vi "MS-200 Send Command.vi"(0 "VISA Ref":refnum<visa-resource-name>, 2 "Wait for Reply (T)":bool=TRUE, 7 "Command":string, 11 "Error In":errorcluster) -> (4 "VISA Ref Dup":refnum<visa-resource-name>, 8 "Reply":string, 13 "Cmd Success":bool, 15 "Error Out":errorcluster)   [LabVIEW 2020]
uses:
  <vilib>/Utility/error.llb/whitespace.ctl
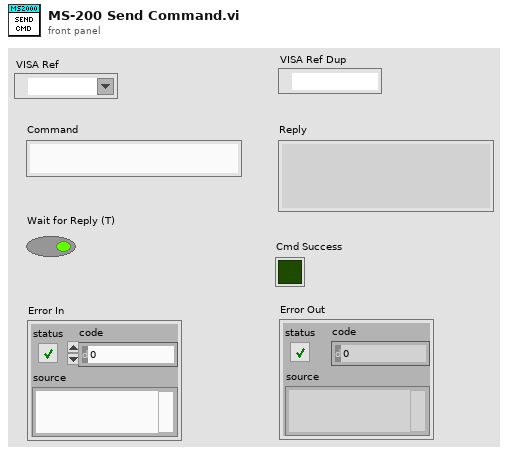
[diagram p1: front panel]
types:
  T1 = typedef "whitespace.ctl" = u16
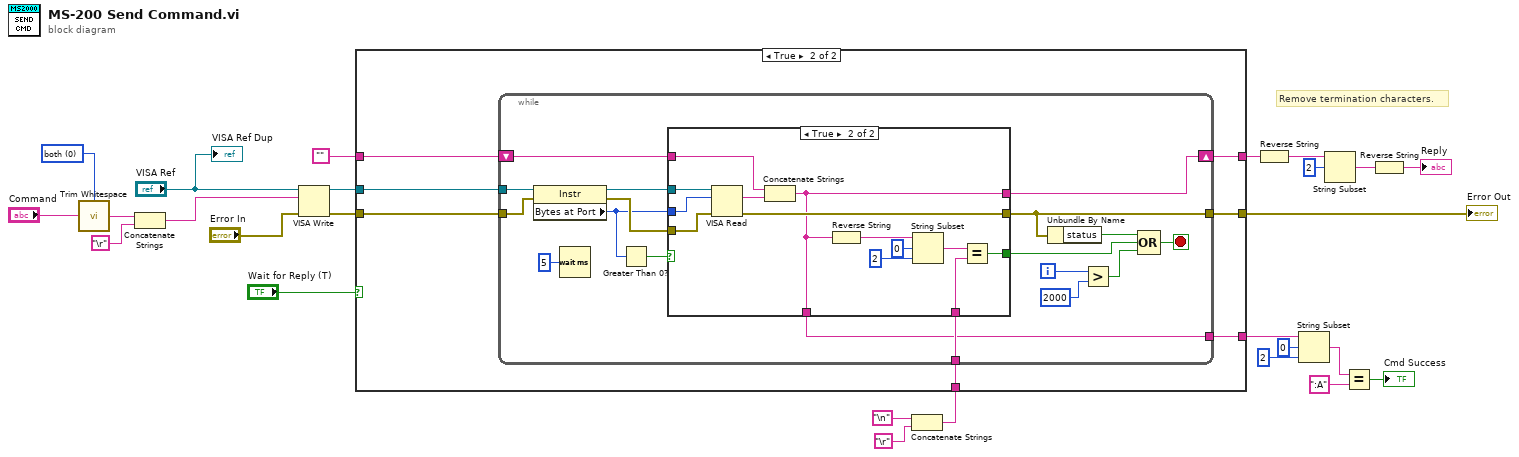
[diagram p0: block diagram]
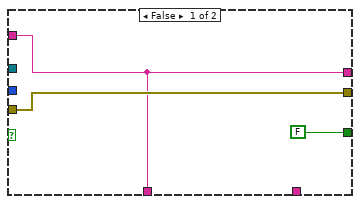
[diagram p3: hidden frame]
diagram:
  w25 = T1 0 items=["both", "start of string", "end of string"] ("location (both)")
  # "Remove termination characters."
  n1 = call <vilib>:"Trim Whitespace.vi"("string"="Command", "location (both)"=w25) -> ("trimmed string"=w24:string)
  n2 = Concatenate Strings(w24, "\r") -> (w23:string)
  n3 = VISA Write(VISA resource name="VISA Ref", write buffer=w23, error in (no error)="Error In") -> (VISA resource name out=w22:refnum<visa-resource-name>, error out=w21:errorcluster)  [unwired: 1 out]
  n4 = Concatenate Strings("\n", "\r") -> (w6:string)
  n5 = case shown="True" "Wait for Reply (T)" {
    tunnel: w22 -> [_ w31]
    tunnel: w21 -> [w28 w30]
    tunnel: "" -> [w27 w35]
    tunnel: [w27 w34] -> w2
    tunnel: [w28 w33] -> w17
    tunnel: w6 -> [_ w32]
    tunnel: [w27 w29] -> w15
    frame False {
    }
    frame True {
      n6 = while {
        tunnel: w31 -> [w53]
        tunnel: w30 -> [w52]
        shift-right: [w41] -> w34
        shift-left: w35 -> [w42]
        tunnel: [w38] -> w33
        tunnel: w32 -> [w37]
        tunnel: [w36] -> w29
        i -> [w51]
        stop <- w48 stop-if-true
        n7 = property class="Instr"(reference=w53, error in=w52) -> (reference out=w44:refnum<visa-resource-name>, error out=w45:errorcluster, "Bytes at Port"=w43:u32)
        n8 = Wait (ms)(milliseconds to wait=u32 5) -> ()  [unwired: 1 out]
        n9 = Greater Than 0?(x=w43) -> (x > 0?=w46:bool)
        n10 = case shown="True" w46 {
          tunnel: w45 -> [w56 w68]
          tunnel: w44 -> [_ w69]
          tunnel: w43 -> [_ w67]
          tunnel: w42 -> [w54 w66]
          tunnel: [w54 w57] -> w41
          tunnel: [w56 w64] -> w38
          tunnel: [FALSE w60] -> w39
          tunnel: w37 -> [_ w59]
          tunnel: [w54 w57] -> w36
          frame False {
          }
          frame True {
            n11 = VISA Read(VISA resource name=w69, byte count=w67, error in (no error)=w68) -> (read buffer=w65:string, error out=w64:errorcluster)  [unwired: 2 out]
            n12 = Concatenate Strings(w66, w65) -> (w57:string)
            n13 = Reverse String(1:w57) -> (0:w58:string)
            n14 = String Subset(string=w58, offset (0)=0, length (rest)=2 ("length (rest)")) -> (substring=w61:string)
            n15 = Equal?(x=w61, y=w59) -> (x = y?=w60:bool)
          }
        }
        n16 = Unbundle By Name(w38) -> ("status"=w40:bool)
        n17 = Greater?(x=w51, y=2000) -> (0:w49:bool)
        n18 = Compound Arithmetic op=OR(w40, w39, w49) -> (w48:bool)
      }
    }
  }
  "Error Out" <- w17
  n19 = Reverse String(1:w2) -> (0:w5:string)
  n20 = String Subset(string=w15, offset (0)=0, length (rest)=2 ("length (rest)")) -> (substring=w12:string)
  n21 = String Subset(string=w5, offset (0)=2) -> (substring=w3:string)  [unwired: 1 in]
  n22 = Equal?(x=w12, y=":A") -> (x = y?=→"Cmd Success":bool)
  n23 = Reverse String(1:w3) -> (0:→"Reply":string)
  "VISA Ref Dup" <- "VISA Ref"
